vi "Funnel_Test.vi"(11 "Joystick Controls":T1) -> ()   [LabVIEW 2020]
uses:
  Utility VIs/Joystick_Controls.ctl
  Subsystems/Funnel/Funnel_Cluster.ctl
  Subsystems/Funnel/Control_States_Funnel.ctl
  Globals/Funnel_global.vi
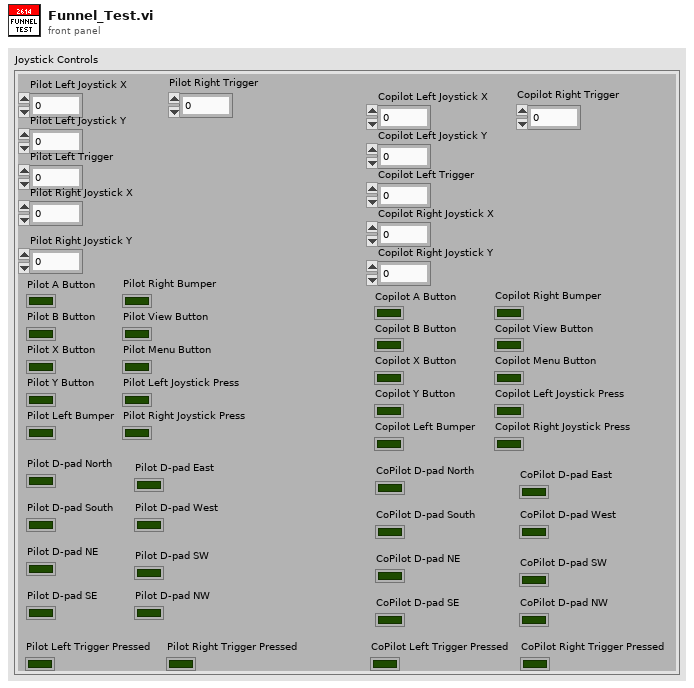
[diagram p1: front panel]
types:
  T1 = typedef "Joystick_Controls.ctl" = cluster{"Pilot Left Joystick X":dbl, "Pilot Left Joystick Y":dbl, "Pilot A Button":bool, "Pilot B Button":bool, "Pilot X Button":bool, "Pilot Y Button":bool, "Pilot Left Bumper":bool, "Pilot Right Bumper":bool, "Pilot View Button":bool, "Pilot Menu Button":bool, "Pilot Left Joystick Press":bool, "Pilot Right Joystick Press":bool, "Pilot Left Trigger":dbl, "Pilot Right Joystick X":dbl, "Pilot Right Joystick Y":dbl, "Pilot Right Trigger":dbl, "Copilot Left Joystick X":dbl, "Copilot Left Joystick Y":dbl, "Copilot A Button":bool, "Copilot B Button":bool, "Copilot X Button":bool, "Copilot Y Button":bool, "Copilot Left Bumper":bool, "Copilot Right Bumper":bool, "Copilot View Button":bool, "Copilot Menu Button":bool, "Copilot Left Joystick Press":bool, "Copilot Right Joystick Press":bool, "Copilot Left Trigger":dbl, "Copilot Right Joystick X":dbl, "Copilot Right Joystick Y":dbl, "Copilot Right Trigger":dbl, "Pilot D-pad North":bool, "Pilot D-pad South":bool, "Pilot D-pad East":bool, "Pilot D-pad West":bool, "Pilot D-pad NE ":bool, "Pilot D-pad SE":bool, "Pilot D-pad SW":bool, "Pilot D-pad NW":bool, "CoPilot D-pad North":bool, "CoPilot D-pad South":bool, "CoPilot D-pad East":bool, "CoPilot D-pad West":bool, "CoPilot D-pad NE":bool, "CoPilot D-pad SE":bool, "CoPilot D-pad SW":bool, "CoPilot D-pad NW":bool, "Pilot Left Trigger Pressed":bool, "Pilot Right Trigger Pressed":bool, "CoPilot Left Trigger Pressed":bool, "CoPilot Right Trigger Pressed":bool}
  T2 = typedef "Funnel_Cluster.ctl" = cluster{"Control States":T3, "Throttle":dbl}
  T3 = typedef "Control_States_Funnel.ctl" = enum16{"No_Op", "Manual_Op"}
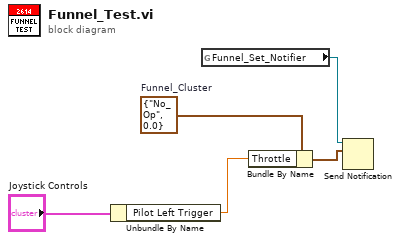
[diagram p0: block diagram]
diagram:
  w4 = T2 {"Control States"=enum."No_Op", "Throttle"=0.0}  # Funnel_Cluster
  n1 = Unbundle By Name("Joystick Controls") -> ("Pilot Left Trigger"=w3:dbl)
  n2 = global read "Funnel_global.vi" "Funnel_Set_Notifier"() -> (w1:refnum<notifier>)
  n3 = Bundle By Name(cluster=w4, "Throttle"=w3) -> (w2:T2)
  n4 = Send Notification(notification=w2, notifier=w1) -> ()  [unwired: 1 in, 2 out]
